vi "Define_Indicies_Crossconnected_Displacements-1.vi"(0 "[IN] Index of Track With \nOther Problem Point \"111\"":i32, 1 "[IN] Index of Other Problem \nPoint \"111\" Inside Track":i32, 2 "[IN] Index of Track with First\n Problem Point":i32, 3 "[IN] Index of First Pro\nblem Point Inside Track":i32, 5 "[IN] The other point for\n crossconnection found":bool, 7 "[IN] Index for initial point":i32, 9 "[IN] Index for other point":i32, 11 "[IN] Index of connected tra\ncks with initial problem point":i32[](array[numeric]), 12 "[IN] Index of connected points \nwith initial point inside the track":i32[](array[numeric]), 13 "[IN] Index of connected trac\nks with other problem point":i32[](array[numeric]), 14 "[IN] Index of connected points \nwith other point inside the track":i32[](array[numeric])) -> (8 "[OUT] Indicies of Cross\nconnected Points":i32[](array[numeric]))   [LabVIEW 2013]
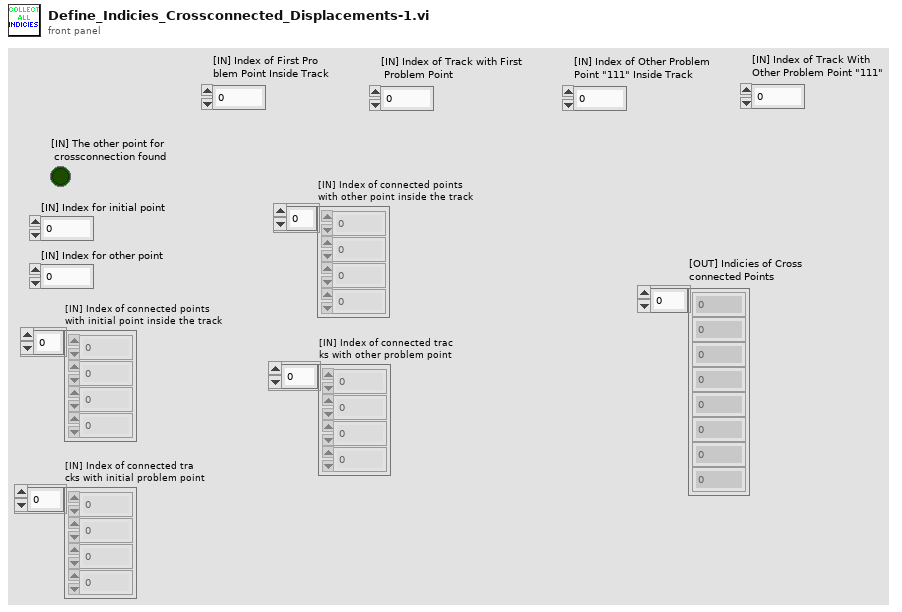
[diagram p1: front panel]
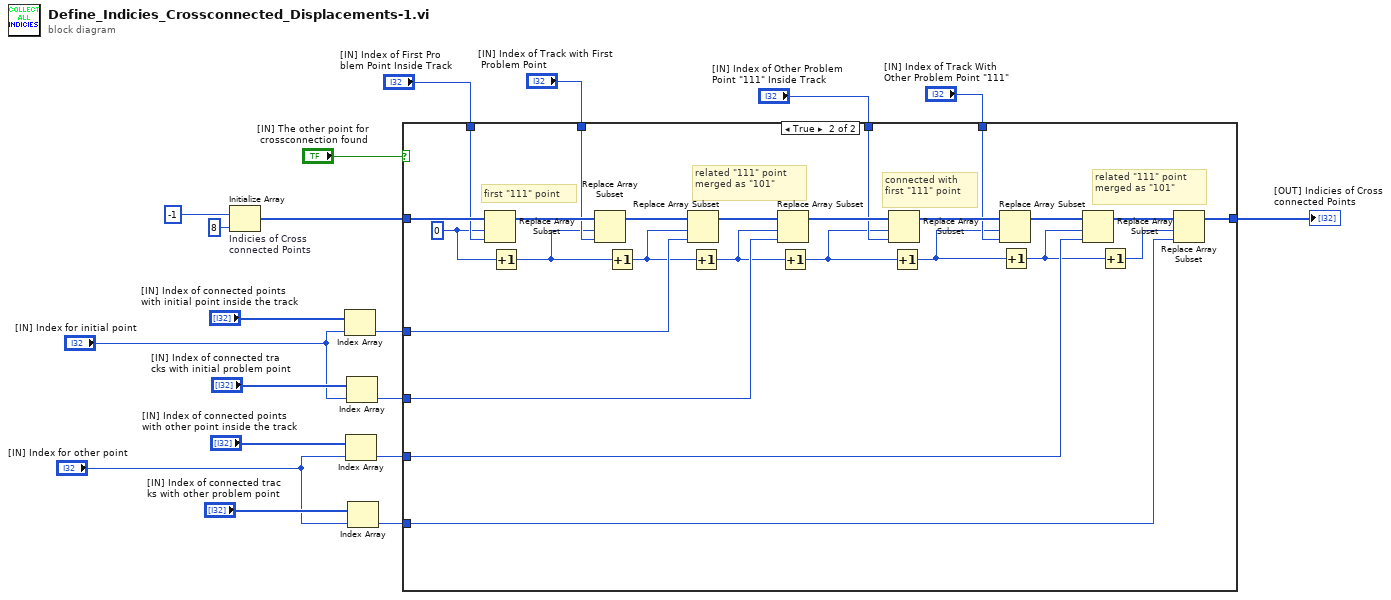
[diagram p0: block diagram]
diagram:
  n1 = Initialize Array "Indicies of Cross\nconnected Points"(-1, 8 ("dimension size")) -> (w16:i32[])
  n2 = Index Array(array="[IN] Index of connected points \nwith initial point inside the track", index="[IN] Index for initial point") -> (element=w10:i32)
  n3 = Index Array(array="[IN] Index of connected points \nwith other point inside the track", index="[IN] Index for other point") -> (element=w3:i32)
  n4 = Index Array(array="[IN] Index of connected tra\ncks with initial problem point", index="[IN] Index for initial point") -> (element=w9:i32)
  n5 = Index Array(array="[IN] Index of connected trac\nks with other problem point", index="[IN] Index for other point") -> (element=w2:i32)
  n6 = case shown="True" "[IN] The other point for\n crossconnection found" {
    tunnel: w16 -> [w20 w45]
    tunnel: "[IN] Index of First Pro\nblem Point Inside Track" -> [_ w44]
    tunnel: "[IN] Index of Track with First\n Problem Point" -> [_ w41]
    tunnel: w10 -> [_ w39]
    tunnel: w9 -> [_ w35]
    tunnel: "[IN] Index of Other Problem \nPoint \"111\" Inside Track" -> [_ w33]
    tunnel: "[IN] Index of Track With \nOther Problem Point \"111\"" -> [_ w30]
    tunnel: w3 -> [_ w27]
    tunnel: w2 -> [_ w26]
    tunnel: [w20 w21] -> w1
    frame False {
    }
    frame True {
      w42 = 0
      # "connected with\nfirst \"111\" point"
      # "related \"111\" point\nmerged as \"101\""
      # "related \"111\" point\nmerged as \"101\""
      # "first \"111\" point"
      n7 = Replace Array Subset(array=w45, new element=w44, index=w42) -> (w43:i32[])
      n8 = Increment(x=w42) -> (x+1=w38:i32)
      n9 = Replace Array Subset(array=w43, new element=w41, index=w38) -> (w40:i32[])
      n10 = Increment(x=w38) -> (x+1=w36:i32)
      n11 = Replace Array Subset(array=w40, new element=w39, index=w36) -> (w37:i32[])
      n12 = Increment(x=w36) -> (x+1=w32:i32)
      n13 = Replace Array Subset(array=w37, new element=w35, index=w32) -> (w34:i32[])
      n14 = Increment(x=w32) -> (x+1=w29:i32)
      n15 = Replace Array Subset(array=w34, new element=w33, index=w29) -> (w31:i32[])
      n16 = Increment(x=w29) -> (x+1=w24:i32)
      n17 = Replace Array Subset(array=w31, new element=w30, index=w24) -> (w28:i32[])
      n18 = Increment(x=w24) -> (x+1=w23:i32)
      n19 = Replace Array Subset(array=w28, new element=w27, index=w23) -> (w25:i32[])
      n20 = Increment(x=w23) -> (x+1=w22:i32)
      n21 = Replace Array Subset(array=w25, new element=w26, index=w22) -> (w21:i32[])
    }
  }
  "[OUT] Indicies of Cross\nconnected Points" <- w1
